vi "Clear Votes.vi"(11 "map in":map{i32, T1}(c390)) -> (3 "map out":map{i32, T1}(c390))   [LabVIEW 2019]
doc: "Clears the voters ballot."
uses:
  SubVIs/Voter Info.ctl
  <vilib>/Utility/miscctls.llb/LVMapReplaceAction.ctl
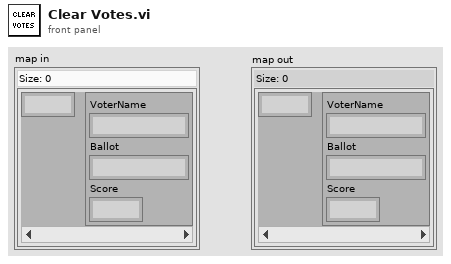
[diagram p1: front panel]
types:
  T1 = typedef "Voter Info.ctl" = cluster{"VoterName":string, "Ballot":string, "Score":i32}
  T2 = typedef "LVMapReplaceAction.ctl" = enum32{"Modify Entry only if found", "Add or Modify Entry", "Delete Entry"}
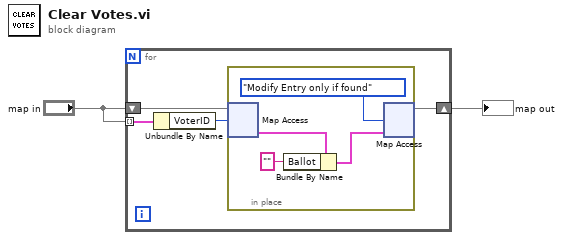
[diagram p0: block diagram]
diagram:
  n1 = for {
    shift-right: [w5] -> w2
    shift-left: "map in" -> [w6]
    tunnel: "map in" -> [w4] mode=indexing
    n2 = Unbundle By Name(w4) -> ("VoterID"=w3:i32)
    n3 = in-place {
      n4 = in-place-map #1(w6, w3) -> (w10:T1)  [unwired: 1 in, 1 out]
      n5 = Bundle By Name(cluster=w10, "Ballot"="") -> (w8:T1)
      n6 = in-place-map #1(w8, LVMapReplaceAction."Modify Entry only if found" ("action")) -> (w5:map{i32, T1})  [unwired: 2 out]
    }
  }
  "map out" <- w2
